vi "Linear_fit_coefficientsph.vi"(0 "XY Graph":cluster{dbl[], dbl[]}[](graph), 1 "Template":path=path "/G4_2_HD/Users/paulhayden/Documents/Projects/Hong Roughness/XW data/XW_Corr.tpt") -> (2 "Saved Automatically?":bool, 3 "Tex Info String":string, 4 "Plot data file":path)   [LabVIEW 2010]
uses:
  Results_plotter_Global.vi
  <vilib>/Analysis/NI_AALPro.lvlib
panel:
  out "intercept":dbl format="%.4f"
  out "slope":dbl format="%.4f"
  out "Current filename index":i32
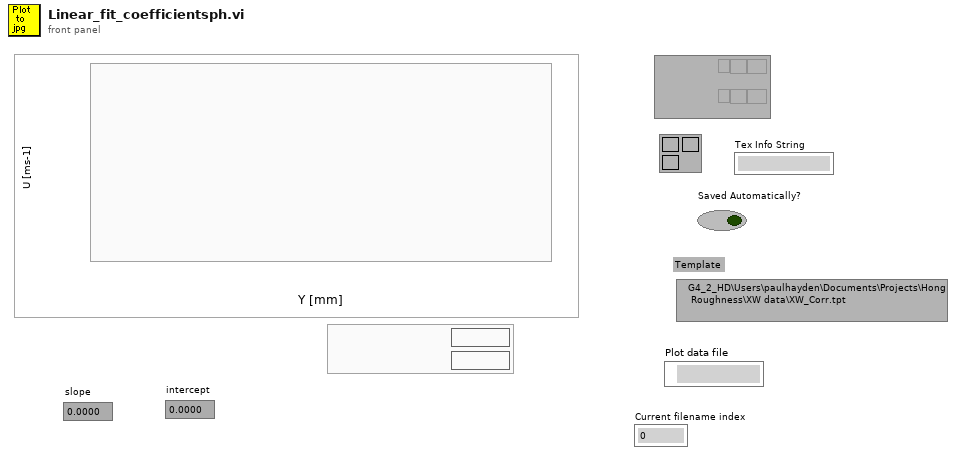
[diagram p1: front panel]
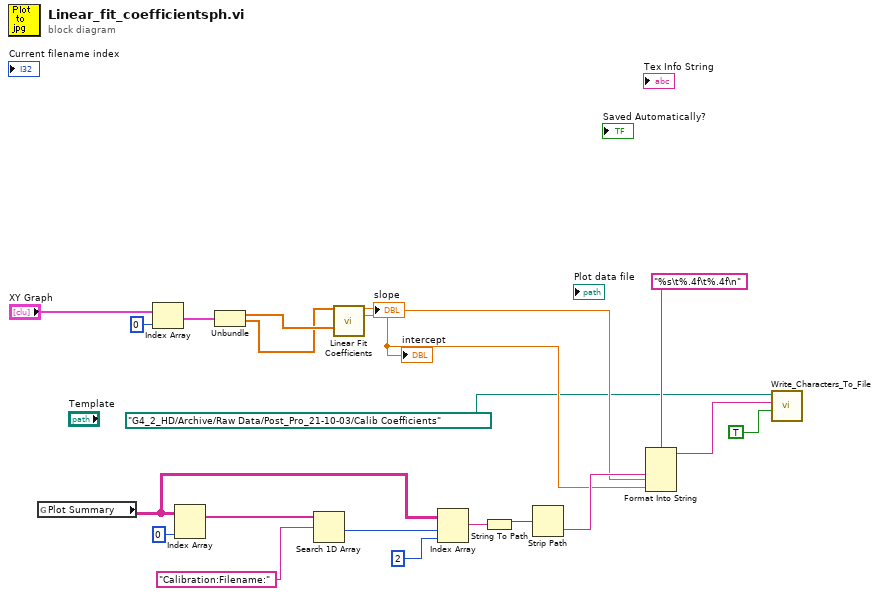
[diagram p0: block diagram]
diagram:
  n1 = global read "Results_plotter_Global.vi" "Plot Summary"() -> (w12:string[][])
  n2 = Index Array(array="XY Graph", index=0) -> (element=w18:cluster{dbl[], dbl[]})
  n3 = Index Array(array=w12, index (col)=0 ("disabled index (col)")) -> (element=w13:string[])  [unwired: 1 in]
  n4 = Unbundle(w18) -> (w17:dbl[], w16:dbl[])
  n5 = Search 1D Array(1D array=w13, element="Calibration:Filename:") -> (index of element=w11:i32)  [unwired: 1 in]
  n6 = call <vilib>:"Linear Fit Coefficients.vi"("Y"=w16, "X"=w17) -> ("slope"=w6:dbl, "intercept"=w5:dbl)  [unwired: 11 in, 1 out]
  "slope" <- w6
  "intercept" <- w5
  n7 = Index Array(array=w12, index (row)=w11, index (col)=2 ("disabled index (col)")) -> (element=w9:string)
  n8 = String To Path(string=w9) -> (path=w8:path)
  n9 = Strip Path(path=w8) -> (name=w7:string)  [unwired: 1 out]
  n10 = Format Into String(format string="%s\t%.4f\t%.4f\n", w7, w6, w5) -> (resulting string=w3:string)  [unwired: 2 in, 1 out]
  n11 = call "Write_Characters_To_File.vi"("file path (dialog if empty)"=path "/G4_2_HD/Archive/Raw Data/Post_Pro_21-10-03/Calib Coefficients" ("Output Filename"), "character string"=w3, "append to file? (new file:F)"=TRUE) -> ()  [unwired: 5 in, 1 out]
